vi "RSZVB Marker x dB Bandwidth ZVR.vi"(7 "x dB Bandwidth (3.0 dB)":dbl=3.0 format="%^.3e", 8 "error in (no error)":errorcluster {"code" format="%.0x"}, 9 "Marker (1)":i32=1, 10 "Channel (Trace) (1)":i32=1, 11 "VISA session":refnum<visa-resource-name>) -> (0 "error out":errorcluster {"code" format="%.0x"}, 3 "dup VISA session":refnum<visa-resource-name>)   [LabVIEW 2011]
doc: "This VI defines the bandfilter level, i.e. the minimum excursion for the bandpass and bandstop peaks.\n\nNote(s):\n\n(1) This VI is ZVR compatible.\n\nRemote-control command(s):\nCALCulate<Ch/Tr>:MARKer<Mk>:FUNCtion:BWIDth <x_dB_Bandwidth>"
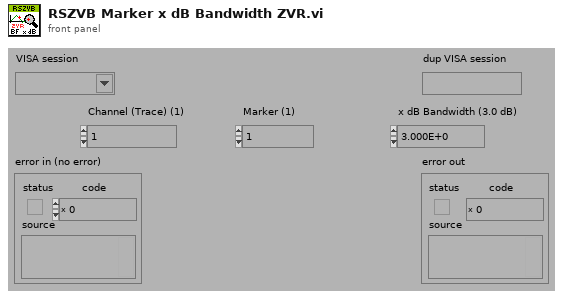
[diagram p1: front panel]
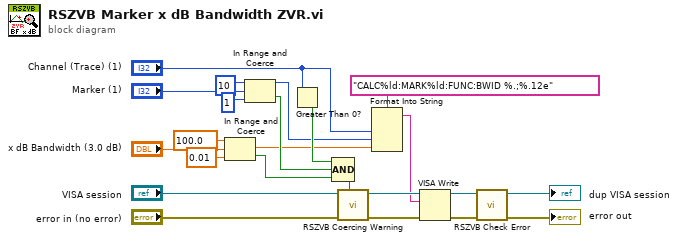
[diagram p0: block diagram]
diagram:
  n1 = In Range and Coerce(upper limit=100.0, x="x dB Bandwidth (3.0 dB)", lower limit=0.01) -> (coerced(x)=w4:dbl, In Range?=w5:bool)
  n2 = In Range and Coerce(upper limit=10, x="Marker (1)", lower limit=1) -> (coerced(x)=w12:i32, In Range?=w13:bool)
  n3 = Greater Than 0?(x="Channel (Trace) (1)") -> (x > 0?=w16:bool)
  n4 = Compound Arithmetic op=AND(w16, w13, w5) -> (w18:bool)
  n5 = call "RSZVB Coercing Warning.vi"("In Range?"=w18, "error in (no error)"="error in (no error)", "VISA session"="VISA session") -> ("error out"=w21:errorcluster, "dup VISA session"=w22:refnum<visa-resource-name>)  [unwired: 7 in]
  n6 = Format Into String(format string="CALC%ld:MARK%ld:FUNC:BWID %.;%.12e", "Channel (Trace) (1)", w12, w4) -> (resulting string=w17:string)  [unwired: 2 in, 1 out]
  n7 = VISA Write(VISA resource name=w22, write buffer=w17, error in (no error)=w21) -> (VISA resource name out=w19:refnum<visa-resource-name>, error out=w20:errorcluster)  [unwired: 1 out]
  n8 = call "RSZVB Check Error.vi"("error in (no error)"=w20, "VISA session"=w19) -> ("error out"=→"error out":errorcluster, "dup VISA session"=→"dup VISA session":refnum<visa-resource-name>)  [unwired: 8 in]
